vi "LaunchServer.vi"(8 "error in (no error)":errorcluster, 11 "TecellaClient in":refnum<class "TecellaClient.lvclass">) -> (0 "error out":errorcluster, 3 "TecellaClient out":refnum<class "TecellaClient.lvclass">)   [LabVIEW 2009, in "TecellaClient.lvclass"]
uses:
  TecellaClient.lvclass
  TecellaClient.lvclass/TecellaClient.ctl
panel:
  out "standard output":string
  in  "Command":string="cmd /k Tecella\n"
  in  "Path":path
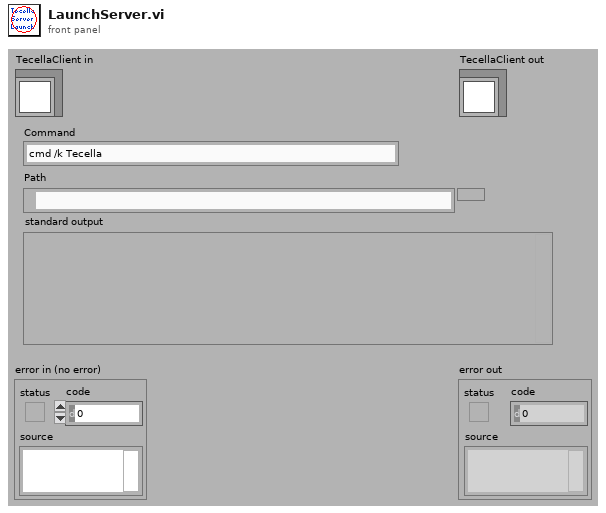
[diagram p1: front panel]
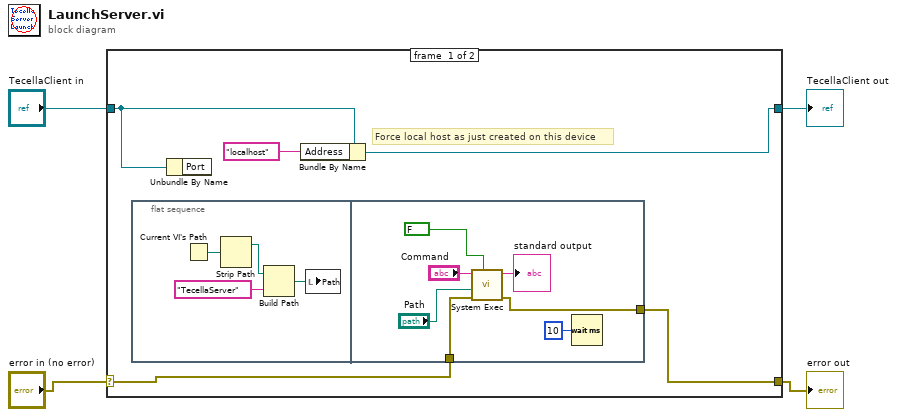
[diagram p0: block diagram]
diagram:
  n1 = case shown="No Error" "error in (no error)" {
    selector: "error in (no error)" -> [w6 w22]
    tunnel: [w5 w22] -> w3
    tunnel: [w7 w21] -> w1
    tunnel: "TecellaClient in" -> [w8 w21]
    frame #0 {
      # "Force local host as just created on this device"
      n2 = flat-sequence {
        tunnel: w6 -> [w16]
        tunnel: [w15] -> w5
        frame #0 {
          n3 = Current VI's Path() -> (path=w10:path)
          n4 = Strip Path(path=w10) -> (stripped path=w12:path)  [unwired: 1 out]
          n5 = Build Path(base path=w12, name or relative path="TecellaServer") -> (appended path=w11:path)
          n6 = local write "Path"(w11) -> ()
        }
        frame #1 {
          n7 = call <vilib>:"System Exec.vi"("wait until completion? (T)"=FALSE, "error in (no error)"=w16, "working directory"="Path", "command line"="Command") -> ("error out"=w15:errorcluster, "standard output"=→"standard output":string)  [unwired: 4 in, 2 out]
          n8 = Wait (ms)(milliseconds to wait=u32 10) -> ()  [unwired: 1 out]
        }
      }
      n9 = Unbundle By Name(w8) -> ()  [unwired: 1 out]
      n10 = Bundle By Name(cluster=w8, "Address"="localhost") -> (w7:refnum<class "TecellaClient.lvclass">)
    }
    frame #1 {
    }
  }
  "error out" <- w3
  "TecellaClient out" <- w1
